vi "CAENHV Deinit System.vi"(8 "error in (no error)":errorcluster, 11 "handle":i32) -> (0 "error out":errorcluster)   [LabVIEW 2014, in "CAENHVWrapper.lvlib"]
doc: "CAENHVLIB_API CAENHVRESULT CAENHV_DeinitSystem(int handle);"
uses:
  CAENHVWrapper.lvlib
  CAENHVWrapper.dll
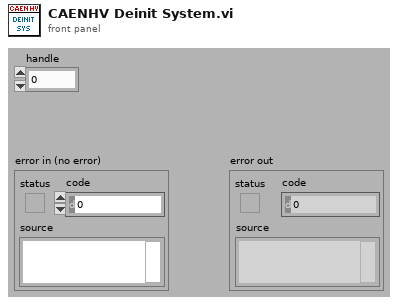
[diagram p1: front panel]
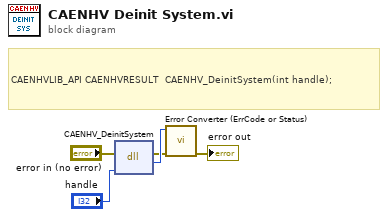
[diagram p0: block diagram]
diagram:
  # "CAENHVLIB_API CAENHVRESULT  CAENHV_DeinitSystem(int handle);"
  n1 = dll-call lib="CAENHVWrapper.*" fn="CAENHV_DeinitSystem"(error in="error in (no error)", "handle"="handle") -> (error out=w2:errorcluster, w3:i32)  [unwired: 3 in, 1 out]
  n2 = call "Error Converter (ErrCode or Status).vi"("error in (no error)"=w2, "error code"=w3) -> ("error out"=→"error out":errorcluster)  [unwired: 9 in]
